vi "moverel.vi"(0 "Xpos":refnum<vi>, 1 "Zpos":refnum<vi>, 2 "Ypos":refnum<vi>, 3 "Z increment":dbl, 5 "VISA resource name":refnum<visa-resource-name>, 6 "Thetapos":refnum<vi>, 7 "X increment":dbl, 9 "Theta on":bool, 11 "error in (no error)":errorcluster, 12 "Y increment":dbl, 13 "Theta inc":dbl) -> (4 "VISA Refnum out":refnum<visa-resource-name>, 15 "error out":errorcluster)   [LabVIEW 2020]
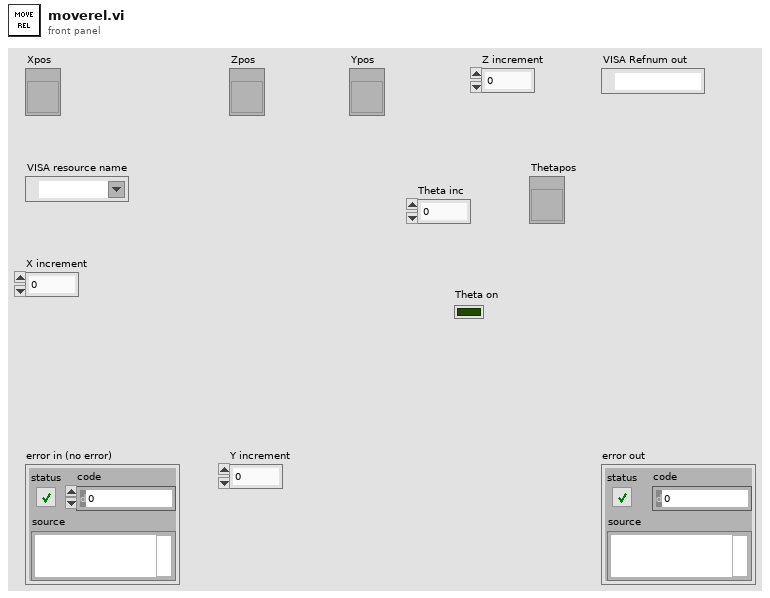
[diagram p1: front panel]
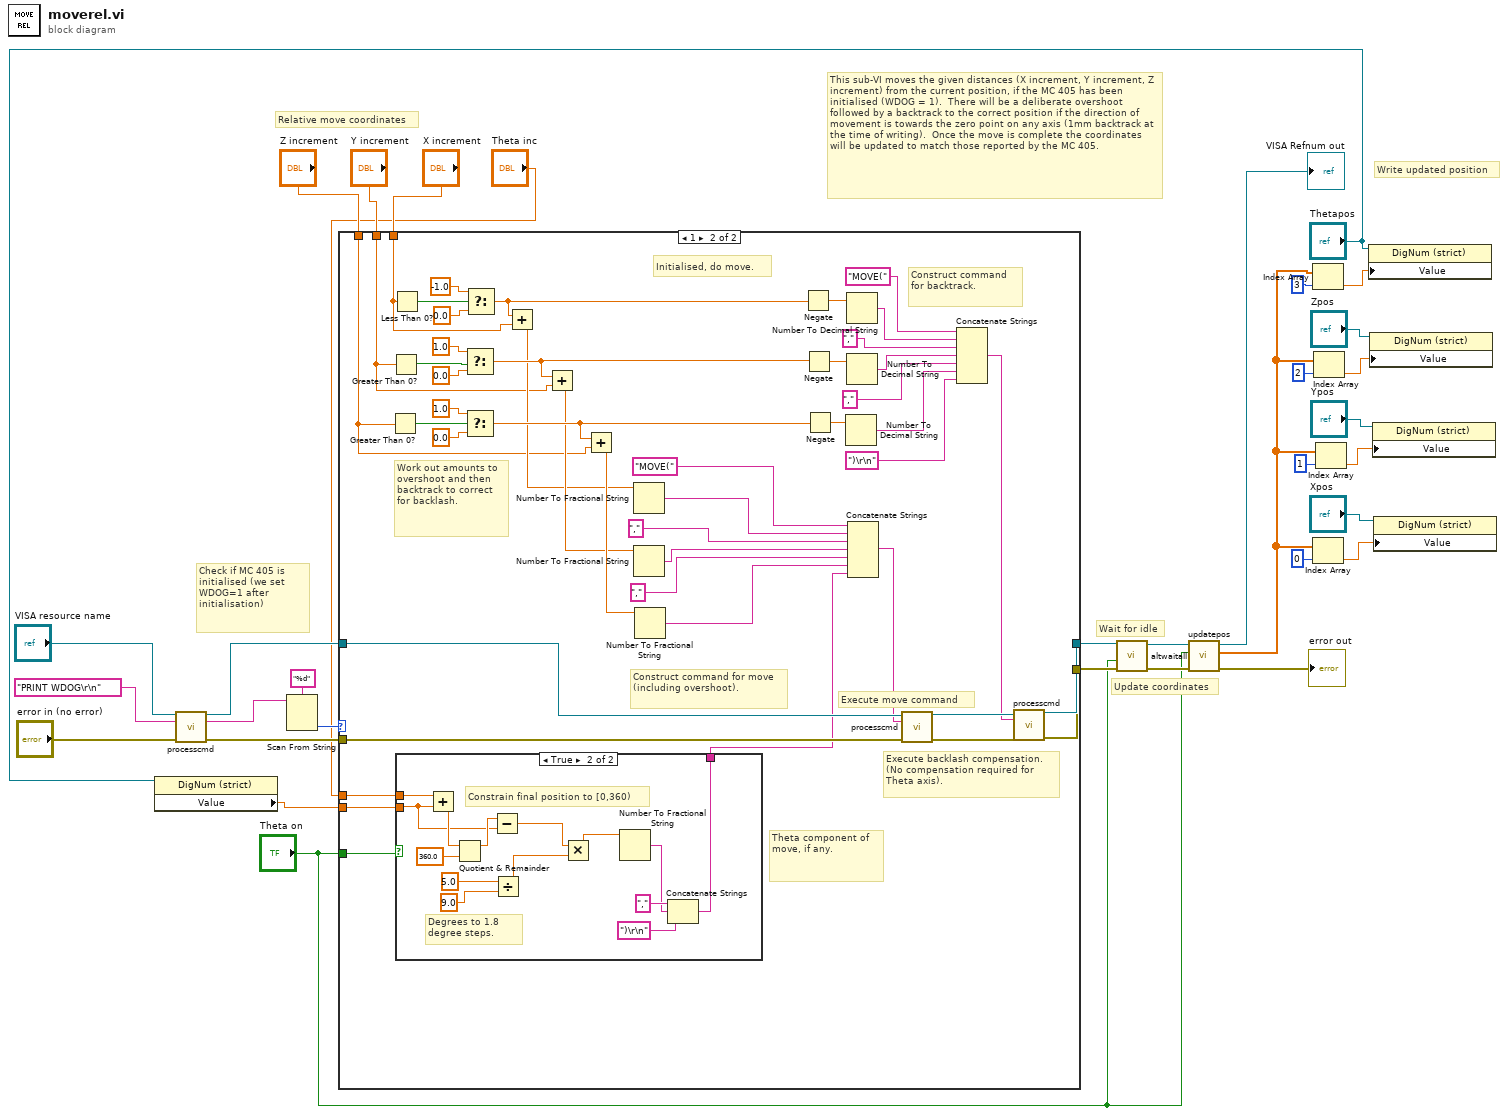
[diagram p0: block diagram]
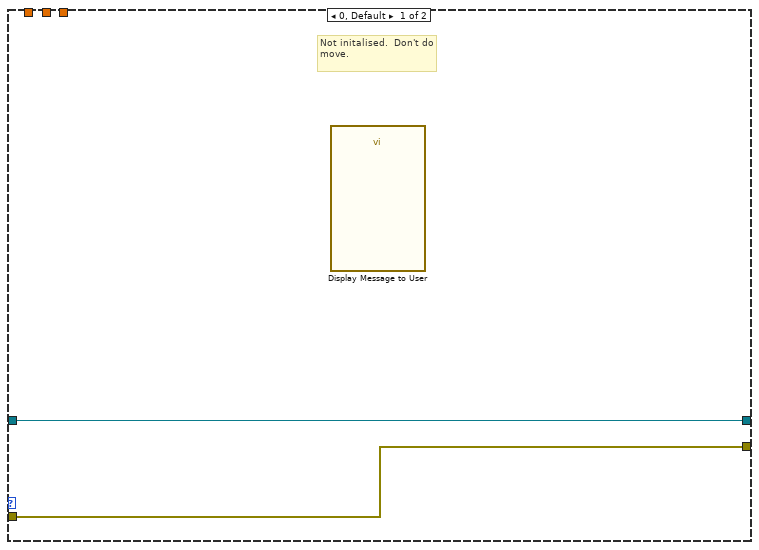
[diagram p2: hidden frame]
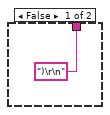
[diagram p3: hidden frame]
diagram:
  # "This sub-VI moves the given distances (X increment, Y increment, Z increment) from the current position, if the MC 405 has been initialised (WDOG = 1).  There will be a deliberate overshoot followed by a backtrack to the correct position if the direction of movement is towards the zero point on any axis (1mm backtrack at the time of writing).  Once the move is complete the coordinates will be updated to match those reported by the MC 405."
  # "Write updated position"
  # "Check if MC 405 is initialised (we set WDOG=1 after initialisation)"
  # "Relative move coordinates"
  # "Update coordinates"
  # "Wait for idle"
  n1 = property class="DigNum (strict)"(reference="Thetapos") -> ("Value"=w1:dbl)  [unwired: 1 in, 2 out]
  n2 = call "processcmd.vi"("VISA Refnum in"="VISA resource name", "write buffer"="PRINT WDOG\r\n", "error in (no error)"="error in (no error)") -> ("VISA Refnum out"=w16:refnum<visa-resource-name>, "read buffer"=w20:string, "error out"=w18:errorcluster)  [unwired: 10 in]
  n3 = Scan From String(format string="%d", input string=w20) -> (output 1=w33:i32)  [unwired: 3 in, 3 out]
  n4 = case shown="1" w33 {
    tunnel: w16 -> [w35 w81]
    tunnel: [w35 w78] -> w17
    tunnel: w18 -> [w34 w80]
    tunnel: [w34 w76] -> w19
    tunnel: "Y increment" -> [_ w41]
    tunnel: "Z increment" -> [_ w42]
    tunnel: "X increment" -> [_ w40]
    tunnel: "Theta on" -> [_ w39]
    tunnel: "Theta inc" -> [_ w38]
    tunnel: w1 -> [_ w36]
    frame 0, Default {
      # "Not initalised.  Don't do move."
      n5 = call "Display Message to User"() -> ()  [unwired: 10 in, 2 out]
    }
    frame 1 {
      # "Theta component of move, if any."
      # "Execute backlash compensation.\n(No compensation required for \nTheta axis)."
      # "Initialised, do move."
      # "Construct command for backtrack."
      # "Construct command for move (including overshoot)."
      # "Work out amounts to overshoot and then backtrack to correct for backlash."
      # "Execute move command"
      n6 = Greater Than 0?(x=w42) -> (x > 0?=w63:bool)
      n7 = Greater Than 0?(x=w41) -> (x > 0?=w62:bool)
      n8 = Less Than 0?(x=w40) -> (x < 0?=w61:bool)
      n9 = case shown="True" w39 {
        tunnel: w38 -> [_ w86]
        tunnel: [")\r\n" ("string") w92] -> w37
        tunnel: w36 -> [_ w84]
        frame False {
        }
        frame True {
          # "Degrees to 1.8 degree steps."
          # "Constrain final position to [0,360)"
          n10 = Add(x=w86, y=w84) -> (x+y=w87:dbl)
          n11 = Quotient & Remainder(x=w87, y=360.0) -> (x-y*floor(x/y)=w85:dbl)  [unwired: 1 out]
          n12 = Subtract(x=w85, y=w84) -> (x-y=w83:dbl)
          n13 = Divide(x=5.0, y=9.0) -> (x/y=w89:dbl)
          n14 = Multiply(x=w83, y=w89) -> (x*y=w88:dbl)
          n15 = Number To Fractional String(number=w88) -> (F-format string=w94:string)  [unwired: 3 in]
          n16 = Concatenate Strings("," ("string"), w94, ")\r\n" ("string")) -> (w92:string)
        }
      }
      n17 = Select(t=1.0, s=w62, f=0.0) -> (s? t:f=w72:dbl)
      n18 = Select(t=1.0, s=w63, f=0.0) -> (s? t:f=w74:dbl)
      n19 = Select(t=-1.0, s=w61, f=0.0) -> (s? t:f=w70:dbl)
      n20 = Add(x=w70, y=w40) -> (x+y=w71:dbl)
      n21 = Add(x=w72, y=w41) -> (x+y=w73:dbl)
      n22 = Add(x=w74, y=w42) -> (x+y=w75:dbl)
      n23 = Number To Fractional String(number=w71) -> (F-format string=w58:string)  [unwired: 3 in]
      n24 = Number To Fractional String(number=w73) -> (F-format string=w59:string)  [unwired: 3 in]
      n25 = Number To Fractional String(number=w75) -> (F-format string=w60:string)  [unwired: 3 in]
      n26 = Negate(x=w70) -> (-x=w64:dbl)
      n27 = Negate(x=w72) -> (-x=w65:dbl)
      n28 = Negate(x=w74) -> (-x=w66:dbl)
      n29 = Number To Decimal String(number=w66) -> (decimal integer string=w69:string)  [unwired: 1 in]
      n30 = Number To Decimal String(number=w64) -> (decimal integer string=w67:string)  [unwired: 1 in]
      n31 = Number To Decimal String(number=w65) -> (decimal integer string=w68:string)  [unwired: 1 in]
      n32 = Concatenate Strings("MOVE(", w58, ",", w59, ",", w60, w37) -> (w44:string)
      n33 = call "processcmd.vi"("VISA Refnum in"=w81, "write buffer"=w44, "error in (no error)"=w80) -> ("VISA Refnum out"=w79:refnum<visa-resource-name>, "error out"=w77:errorcluster)  [unwired: 10 in, 1 out]
      n34 = Concatenate Strings("MOVE(", w67, ",", w68, ",", w69, ")\r\n") -> (w43:string)
      n35 = call "processcmd.vi"("VISA Refnum in"=w79, "write buffer"=w43, "error in (no error)"=w77) -> ("VISA Refnum out"=w78:refnum<visa-resource-name>, "error out"=w76:errorcluster)  [unwired: 10 in, 1 out]
    }
  }
  n36 = call "altwaitall.vi"("error in (no error)"=w19, "Theta enabled"="Theta on", "VISA Refnum in"=w17) -> ("error out"=w21:errorcluster, "VISA Refnum out"=w22:refnum<visa-resource-name>)  [unwired: 7 in]
  n37 = call "updatepos.vi"("error in (no error)"=w21, "Theta enabled"="Theta on", "VISA Refnum in"=w22) -> ("error out"=→"error out":errorcluster, "PosArray"=w4:dbl[], "VISA Refnum out"=→"VISA Refnum out":refnum<visa-resource-name>)  [unwired: 6 in]
  n38 = Index Array(array=w4, index=3) -> (element=w5:dbl)
  n39 = Index Array(array=w4, index=0) -> (element=w25:dbl)
  n40 = Index Array(array=w4, index=2) -> (element=w23:dbl)
  n41 = Index Array(array=w4, index=1) -> (element=w24:dbl)
  n42 = property class="DigNum (strict)"(reference="Thetapos", "Value"=w5) -> ()  [unwired: 1 in, 2 out]
  n43 = property class="DigNum (strict)"(reference="Zpos", "Value"=w23) -> ()  [unwired: 1 in, 2 out]
  n44 = property class="DigNum (strict)"(reference="Ypos", "Value"=w24) -> ()  [unwired: 1 in, 2 out]
  n45 = property class="DigNum (strict)"(reference="Xpos", "Value"=w25) -> ()  [unwired: 1 in, 2 out]
